vi "DoubleFloat (Scalar) to String.vi"(7 "Use System Default Notation (F)":bool, 11 "Value (Double)":dbl format="%#_16g") -> (3 "Value (String)":string)   [LabVIEW 2013, in "OpenScalar.lvlib"]
uses:
  OpenScalar.lvlib
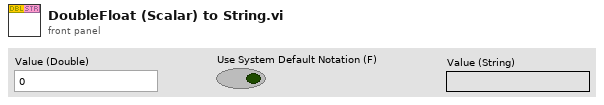
[diagram p1: front panel]
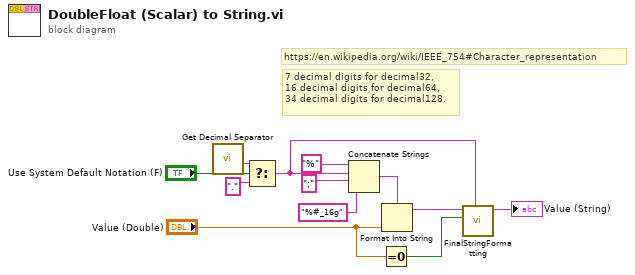
[diagram p0: block diagram]
diagram:
  # "7 decimal digits for decimal32,\n16 decimal digits for decimal64,\n34 decimal digits for decimal128."
  # "https://en.wikipedia.org/wiki/IEEE_754#Character_representation"
  n1 = call "Get Decimal Separator.vi"() -> ("System Decimal separator"=w11:string)  [unwired: 11 in]
  n2 = Select(t=w11, s="Use System Default Notation (F)", f="." ("format string")) -> (s? t:f=w3:string)
  n3 = Concatenate Strings("%" ("format string"), w3, ";" ("regular expression"), "%#_16g" ("format string")) -> (w5:string)
  n4 = Equal To 0?(x="Value (Double)") -> (x = 0?=w1:bool)
  n5 = Format Into String(format string=w5, "Value (Double)") -> (resulting string=w4:string)  [unwired: 2 in, 1 out]
  n6 = call "FinalStringFormatting.vi"("Decimal Notation (.)"=w3, "Equals Zero?"=w1, "String in"=w4) -> ("String out"=→"Value (String)":string)  [unwired: 8 in]
